vi "CRYPIC SHOW FRAME.vi"(10 "tFrame":T2) -> (2 "tFrame_Out":T2)   [LabVIEW 2013]
uses:
  <vilib>/Utility/miscctls.llb/LVRectTypeDef.ctl
  CRYStepSetup/CRYStepSetup Global.vi
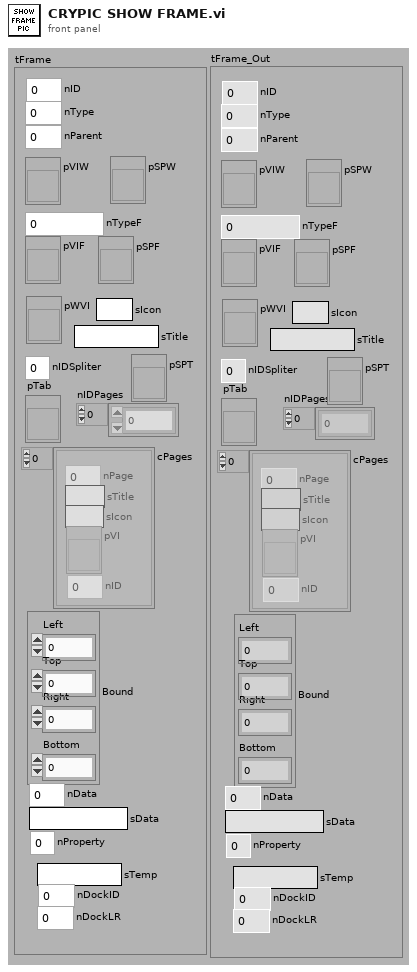
[diagram p1: front panel]
types:
  T1 = typedef "LVRectTypeDef.ctl" = cluster{"Left":i16, "Top":i16, "Right":i16, "Bottom":i16}
  T2 = cluster{"nType":i32, "nParent":i32, "pVIW":refnum<vi>, "pSPW":refnum<vi>, "nTypeF":i32, "pVIF":refnum<vi>, "pSPF":refnum<vi>, "nIDSpliter":i32, "nProperty":i32, "Bound":T1, "nID":i32, "nData":i32, "sData":string, "pWVI":refnum<vi>, "sTitle":string, "cPages":cluster{"nPage":i32, "sTitle":string, "sIcon":string, "pVI":refnum<vi>, "nID":i32}[], "pTab":refnum<vi>, "nIDPages":i32[], "pSPT":refnum<vi>, "sTemp":string, "nDockID":i32, "nDockLR":i32, "sIcon":string}
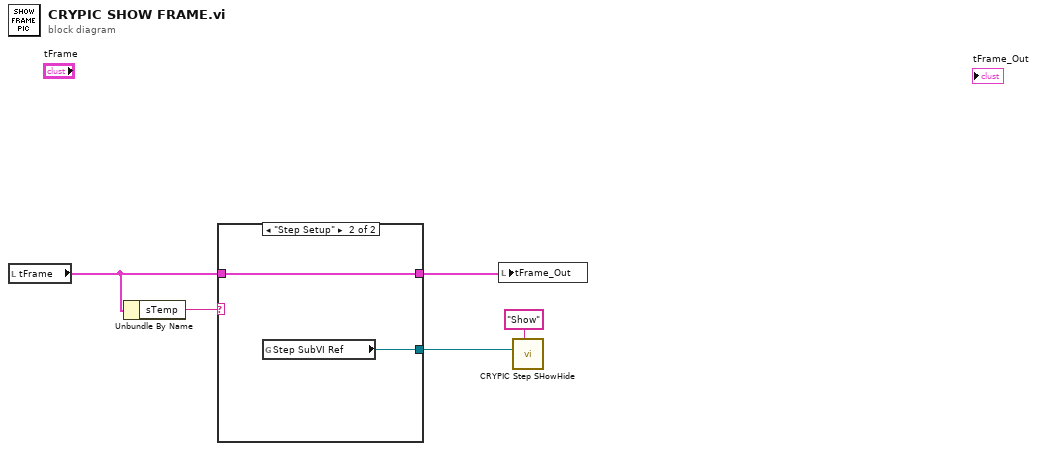
[diagram p0: block diagram]
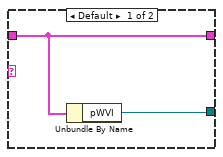
[diagram p2: hidden frame]
diagram:
  n1 = local read "tFrame"() -> (w5:T2)
  n2 = Unbundle By Name(w5) -> ("sTemp"=w4:string)
  n3 = case shown="\"Step Setup\"" w4 {
    tunnel: w5 -> [w7 w9]
    tunnel: [w7 w9] -> w1
    tunnel: [w6 w8] -> w3
    frame Default {
      n4 = Unbundle By Name(w7) -> ("pWVI"=w6:refnum<vi>)
    }
    frame "Step Setup" {
      n5 = global read "CRYStepSetup Global.vi" "Step SubVI Ref"() -> (w8:refnum<vi>)
    }
  }
  n6 = local write "tFrame_Out"(w1) -> ()
  n7 = call "CRYPIC Step SHowHide.vi"("sAction"="Show", "VIRef"=w3) -> ()  [unwired: 10 in]
